vi "Two Lockins.vi"(8 "error in (no error)":errorcluster, 11 "Two Lockins in":refnum<class "Two Lockins.lvclass">) -> (0 "error out":errorcluster, 3 "Two Lockins out":refnum<class "Two Lockins.lvclass">)   [LabVIEW 2017, in "Two Lockins.lvclass"]
uses:
  Two Lockins.lvclass
  C:/LabVIEW-programs/Instruments/Utility Classes/Readable/Readable.lvclass
  Two Lockins.lvclass/Two Lockins.ctl
  Global/GPIB Numbers.vi
  Utility Classes/Readable/Readable.lvclass
panel:
  out "Status":string
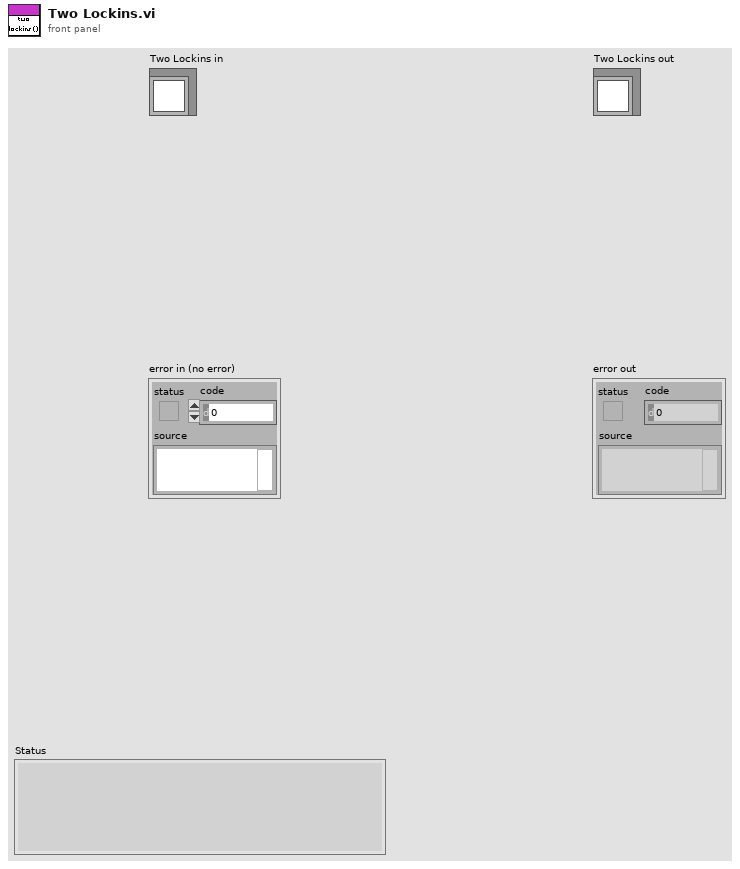
[diagram p1: front panel]
types:
  T1 = typedef "GPIB Type Def.ctl" = cluster{"Name":string, "bus":dbl, "GPIB":dbl, "GPIB as string":string, "byte":i32, "VISA Resource Name":refnum<visa-resource-name>}
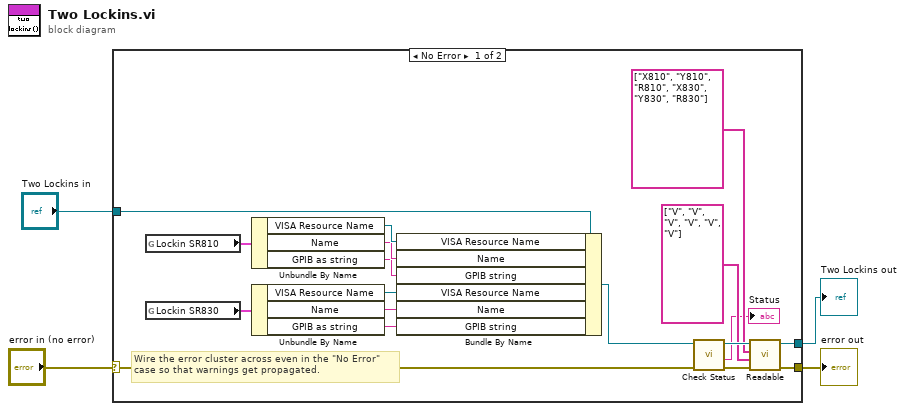
[diagram p0: block diagram]
diagram:
  n1 = case shown="No Error" "error in (no error)" {
    selector: "error in (no error)" -> [w12 w24]
    tunnel: [w6 w24] -> w3
    tunnel: [w10 w23] -> w1
    tunnel: "Two Lockins in" -> [w20 w23]
    frame No Error {
      # "Wire the error cluster across even in the \"No Error\"\ncase so that warnings get propagated."
      n2 = global read "GPIB Numbers.vi" "Lockin SR810"() -> (w22:T1)
      n3 = global read "GPIB Numbers.vi" "Lockin SR830"() -> (w21:T1)
      n4 = Unbundle By Name(w22) -> ("VISA Resource Name"=w19:refnum<visa-resource-name>, "Name"=w18:string, "GPIB as string"=w17:string)
      n5 = Unbundle By Name(w21) -> ("VISA Resource Name"=w16:refnum<visa-resource-name>, "Name"=w15:string, "GPIB as string"=w14:string)
      n6 = Bundle By Name(cluster=w20, "VISA Resource Name"=w19, "Name"=w18, "GPIB string"=w17, "VISA Resource Name"=w16, "Name"=w15, "GPIB string"=w14) -> (w13:refnum<class "Two Lockins.lvclass">)
      n7 = call-dynamic "Check Status.vi"("error in (no error)"=w12, "Two Lockins in"=w13) -> ("error out"=w7:errorcluster, "Status"=→"Status":string, "Two Lockins out"=w11:refnum<class "Two Lockins.lvclass">)  [unwired: 6 in, 1 out]
      n8 = call "Readable.vi"("error in (no error)"=w7, "Channel Units"=string[] ["V", "V", "V", "V", "V", "V"], "Channel Names"=string[] ["X810", "Y810", "R810", "X830", "Y830", "R830"], "Readable in"=w11) -> ("error out"=w6:errorcluster, "Readable out"=w10:refnum<class "Two Lockins.lvclass">)  [unwired: 6 in]
    }
    frame Error {
    }
  }
  "error out" <- w3
  "Two Lockins out" <- w1
